vi "Read SPI.vi"(8 "error in (no error)":errorcluster, 11 "LINX-ADS1015 in":refnum<class "LINX-ADS1256.lvclass">) -> (0 "error out":errorcluster, 2 "LINX SPI":refnum<class "LINX SPI.lvclass">, 3 "LINX-ADS1015 out":refnum<class "LINX-ADS1256.lvclass">)   [LabVIEW 2020, in "LINX-ADS1256.lvclass"]
uses:
  LINX-ADS1256.lvclass
  LINX SPI/LINX SPI.lvclass
  LINX-ADS1256.lvclass/LINX-ADS1256.ctl
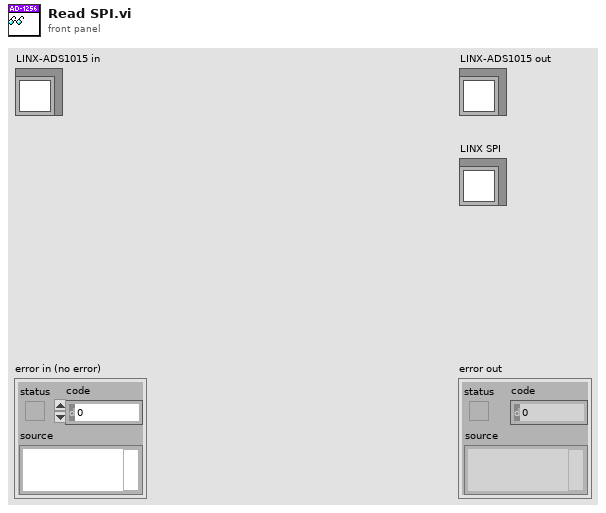
[diagram p1: front panel]
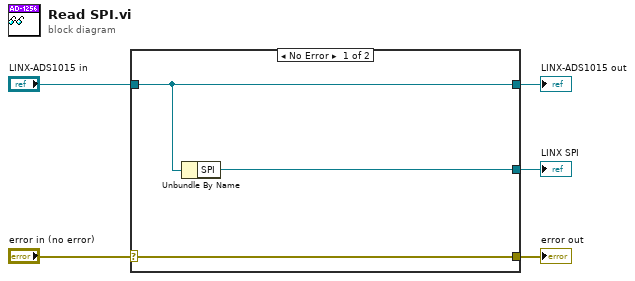
[diagram p0: block diagram]
diagram:
  n1 = case shown="No Error" "error in (no error)" {
    selector: "error in (no error)" -> [w8 w9]
    tunnel: [w8 w9] -> w4
    tunnel: [w7 w10] -> w2
    tunnel: "LINX-ADS1015 in" -> [w7 w10]
    tunnel: [w6 _] -> w1
    frame No Error {
      n2 = Unbundle By Name(w7) -> ("SPI"=w6:refnum<class "LINX SPI.lvclass">)
    }
    frame Error {
    }
  }
  "error out" <- w4
  "LINX-ADS1015 out" <- w2
  "LINX SPI" <- w1
